vi "CaptureImageAtPosition(Async).vi"(6 "timeout in ms (5000)":i32=5000, 8 "error in (no error)":errorcluster, 10 "Coords":T1, 11 "Microscope":refnum<class "Microscope.lvclass">) -> (0 "error out":errorcluster, 2 "buffer":i32, 3 "Microscope out":refnum<class "Microscope.lvclass">)   [LabVIEW 2015, in "Microscope.lvclass"]
doc: "---------------------------------------------------------------\nJKI State Machine Objects™\nhttp://jki.net/state-machine-objects/\nCopyright (C) 2005-2015, JKI <info@jki.net>\nALL RIGHTS RESERVEDJKI State Machine Objects (SMO) 1.0.0.4\nJKI - JKI\nCopyright (c) 2015, JKI"
uses:
  Microscope.lvclass
  XYStage/Typedefs/(real)Coords--Cluster.ctl
  Microscope.lvclass/Microscope.ctl
  Typedefs/PrivateEvents--Microscope.CaptureImageAtPosition.ctl
  XYStage/XYStage.lvclass
panel:
  # "For instructions on how to use the JKI State Machine Objects, examples and video tutorials, visit:\nhttp://jki.net/state-machine-objects/\n\nJKI State Machine Objects™\nhttp://jki.net/state-machine-objects/\nCopyright (C) 2005-2015, JKI <info@jki.net>\nALL RIGHTS RESERVED"
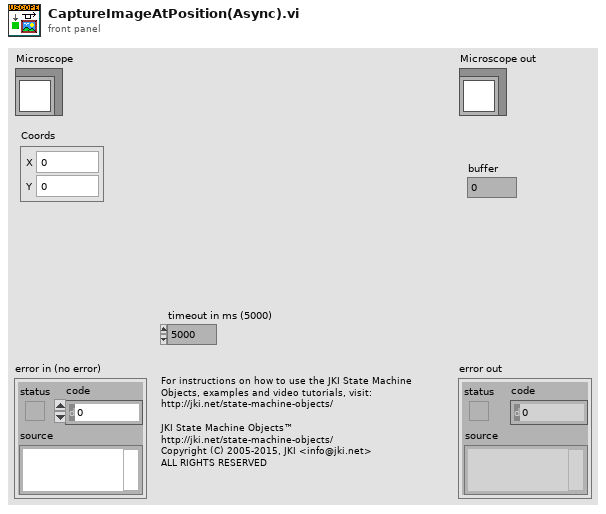
[diagram p1: front panel]
types:
  T1 = typedef "XYStage.lvclass/(real)Coords--Cluster.ctl" = cluster{"X":dbl, "Y":dbl}
  T2 = typedef "Microscope.lvclass/PrivateEvents--Microscope.CaptureImageAtPosition.ctl" = cluster{"Coords":T1, "image notifier":refnum<notifier>, "Move?":bool}
  T3 = typedef "Microscope.lvclass/PrivateData--Ref.ctl" = refnum<data-value>
  T4 = typedef "Microscope.lvclass/PrivateData--Cluster.ctl" = cluster{"Public Events":T5, "Protected Events":T6, "Private Events":T7, "Dependencies":T8, "Configuration":T9}
  T5 = typedef "Microscope.lvclass/PublicEvents--Cluster.ctl" = cluster{"Value Changed":refnum<user-event>, "Initialized":refnum<user-event>}
  T6 = typedef "Microscope.lvclass/ProtectedEvents--Cluster.ctl" = cluster{"placeholder":refnum<user-event>}
  T7 = typedef "Microscope.lvclass/PrivateEvents--Cluster.ctl" = cluster{"New Value":refnum<user-event>, "Initialize":refnum<user-event>, "CaptureImageAtPosition":refnum<user-event>}
  T8 = typedef "Microscope.lvclass/Dependencies--Cluster.ctl" = cluster{"XYStage":refnum<class "XYStage.lvclass">, "Camera":refnum<class "Camera.lvclass">}
  T9 = typedef "Microscope.lvclass/Configuration--Cluster.ctl" = cluster{"XY Stage":string, "Camera":string, "image output folder":path, "filetype":string}
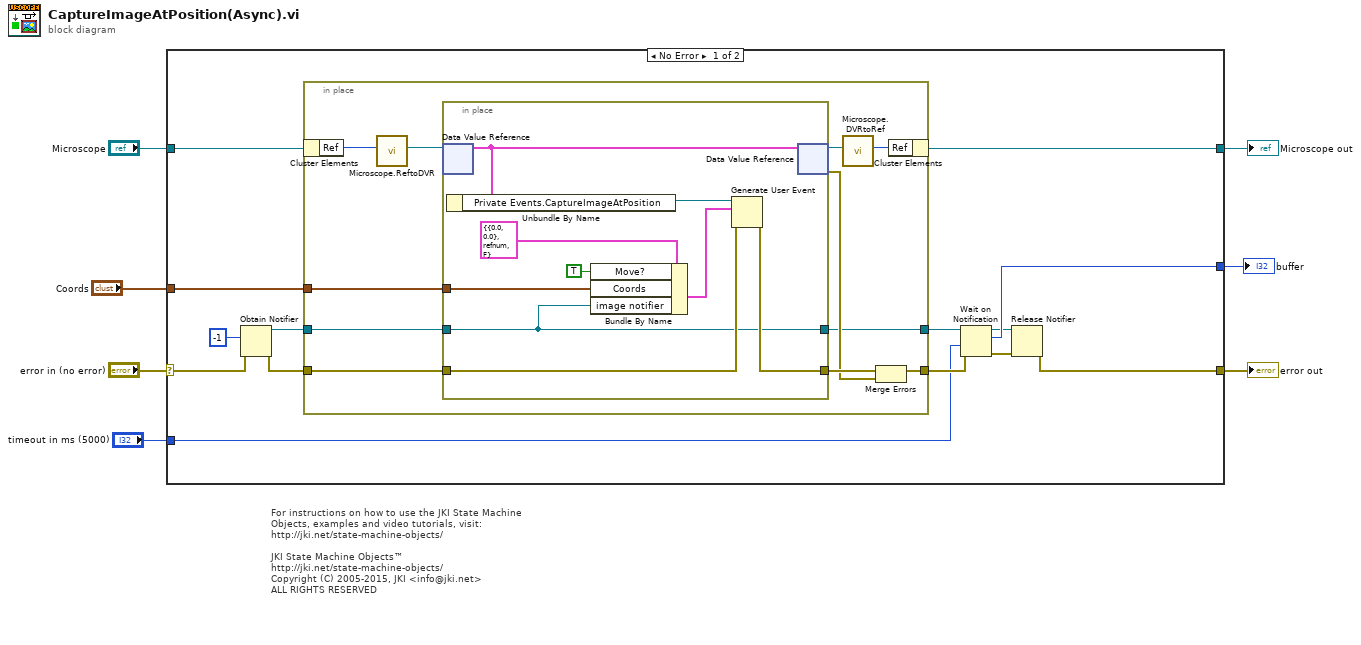
[diagram p0: block diagram]
diagram:
  # "For instructions on how to use the JKI State Machine Objects, examples and video tutorials, visit:\nhttp://jki.net/state-machine-objects/\n\nJKI State Machine Objects™\nhttp://jki.net/state-machine-objects/\nCopyright (C) 2005-2015, JKI <info@jki.net>\nALL RIGHTS RESERVED"
  n1 = case shown="No Error" "error in (no error)" {
    selector: "error in (no error)" -> [w16 w43]
    tunnel: [w10 w43] -> w6
    tunnel: [w20 w42] -> w7
    tunnel: "Microscope" -> [w21 w42]
    tunnel: "Coords" -> [w19 _]
    tunnel: [w12 _] -> w2
    tunnel: "timeout in ms (5000)" -> [w8 _]
    frame No Error {
      n2 = Obtain Notifier(notification data type=-1 ("buffer"), error in (no error)=w16) -> (notifier out=w17:refnum<notifier>, error out=w15:errorcluster)  [unwired: 2 in, 1 out]
      n3 = in-place {
        in-place-border: w15 -> [w32]
        in-place-border: [w29] -> w9
        in-place-border: w19 -> [w24]
        in-place-border: w17 -> [w23]
        in-place-border: [w22] -> w14
        n4 = in-place-cluster #1(w21) -> ("Ref"=w28:u32)
        n5 = call "Microscope.ReftoDVR.vi"("Ref"=w28) -> ("Ref"=w26:T3)  [unwired: 10 in]
        n6 = in-place {
          in-place-border: w32 -> [w39]
          in-place-border: [w38] -> w31
          in-place-border: w24 -> [w36]
          in-place-border: w23 -> [w35]
          in-place-border: [w35] -> w22
          n7 = in-place-dvr #2(w26) -> (w41:T4)  [unwired: 1 out]
          n8 = Unbundle By Name(w41) -> ("Private Events.CaptureImageAtPosition"=w40:refnum<user-event>)
          n9 = Bundle By Name(cluster=T2 {"Coords"={"X"=0.0, "Y"=0.0}, "image notifier"=refnum, "Move?"=FALSE} ("CaptureImageAtPosition"), "Move?"=TRUE, "Coords"=w36, "image notifier"=w35) -> (w34:T2)
          n10 = Generate User Event(user event=w40, event data cluster=w34, error in=w39) -> (error out=w38:errorcluster)  [unwired: 1 in, 1 out]
          n11 = in-place-dvr #2(w41) -> (w27:T3, w30:errorcluster)
        }
        n12 = call "Microscope.DVRtoRef.vi"("Ref"=w27) -> ("Ref"=w25:u32)  [unwired: 10 in]
        n13 = Merge Errors(w31, w30) -> (w29:errorcluster)
        n14 = in-place-cluster #1("Ref"=w25) -> (w20:refnum<class "Microscope.lvclass">)
      }
      n15 = Wait on Notification(notifier=w14, timeout in ms (-1)=w8, error in (no error)=w9) -> (notifier out=w11:refnum<notifier>, notification=w12:i32, error out=w13:errorcluster)  [unwired: 1 in, 1 out]
      n16 = Release Notifier(notifier=w11, error in (no error)=w13) -> (error out=w10:errorcluster)  [unwired: 1 in, 2 out]
    }
    frame Error {
    }
  }
  "error out" <- w6
  "Microscope out" <- w7
  "buffer" <- w2
